vi "RenameVI.vi"(0 "ObjectIn":refnum<class "ClassWriterNative.lvclass">, 1 "VIItemRefIn":refnum<vi>, 2 "RenameOption":T1, 5 "error in (no error)":errorcluster) -> (14 "ObjectOut":refnum<class "ClassWriterNative.lvclass">, 19 "error out":errorcluster)   [LabVIEW 2012, in "ClassWriterNative.lvclass"]
uses:
  <resource>/Framework/Providers/Open_GDS/ClassProviders/Provider_LvNativeClass/ClassWriterNative_class/ClassWriterNative.lvclass
  <resource>/Framework/Providers/Open_GDS/ClassProviders/Provider_BaseClassInterface/ClassWriter_class/RenameViOption.ctl
  <vilib>/picture/picture.llb/imagedata.ctl
  <resource>/Framework/Providers/Open_GDS/ClassProviders/Provider_BaseClassInterface/ClassWriter_class/ClassWriter.lvclass
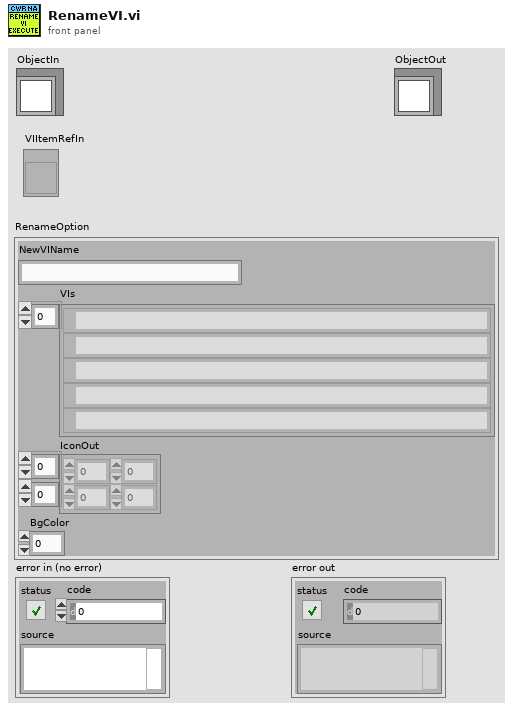
[diagram p1: front panel]
types:
  T1 = typedef "ClassWriter.lvclass/RenameViOption.ctl" = cluster{"NewVIName":string, "VIs":path[], "IconOut":u8[][], "BgColor":u8}
  T2 = cluster{"Counter":i32, "Text":string, "Cancelled":bool, "App Ref":refnum<vi>}
  T3 = typedef "imagedata.ctl" = cluster{"image type":i32, "image depth":i32, "image":u8[], "mask":u8[], "colors":u32[], "Rectangle":cluster{"left":i16, "top":i16, "right":i16, "bottom":i16}}
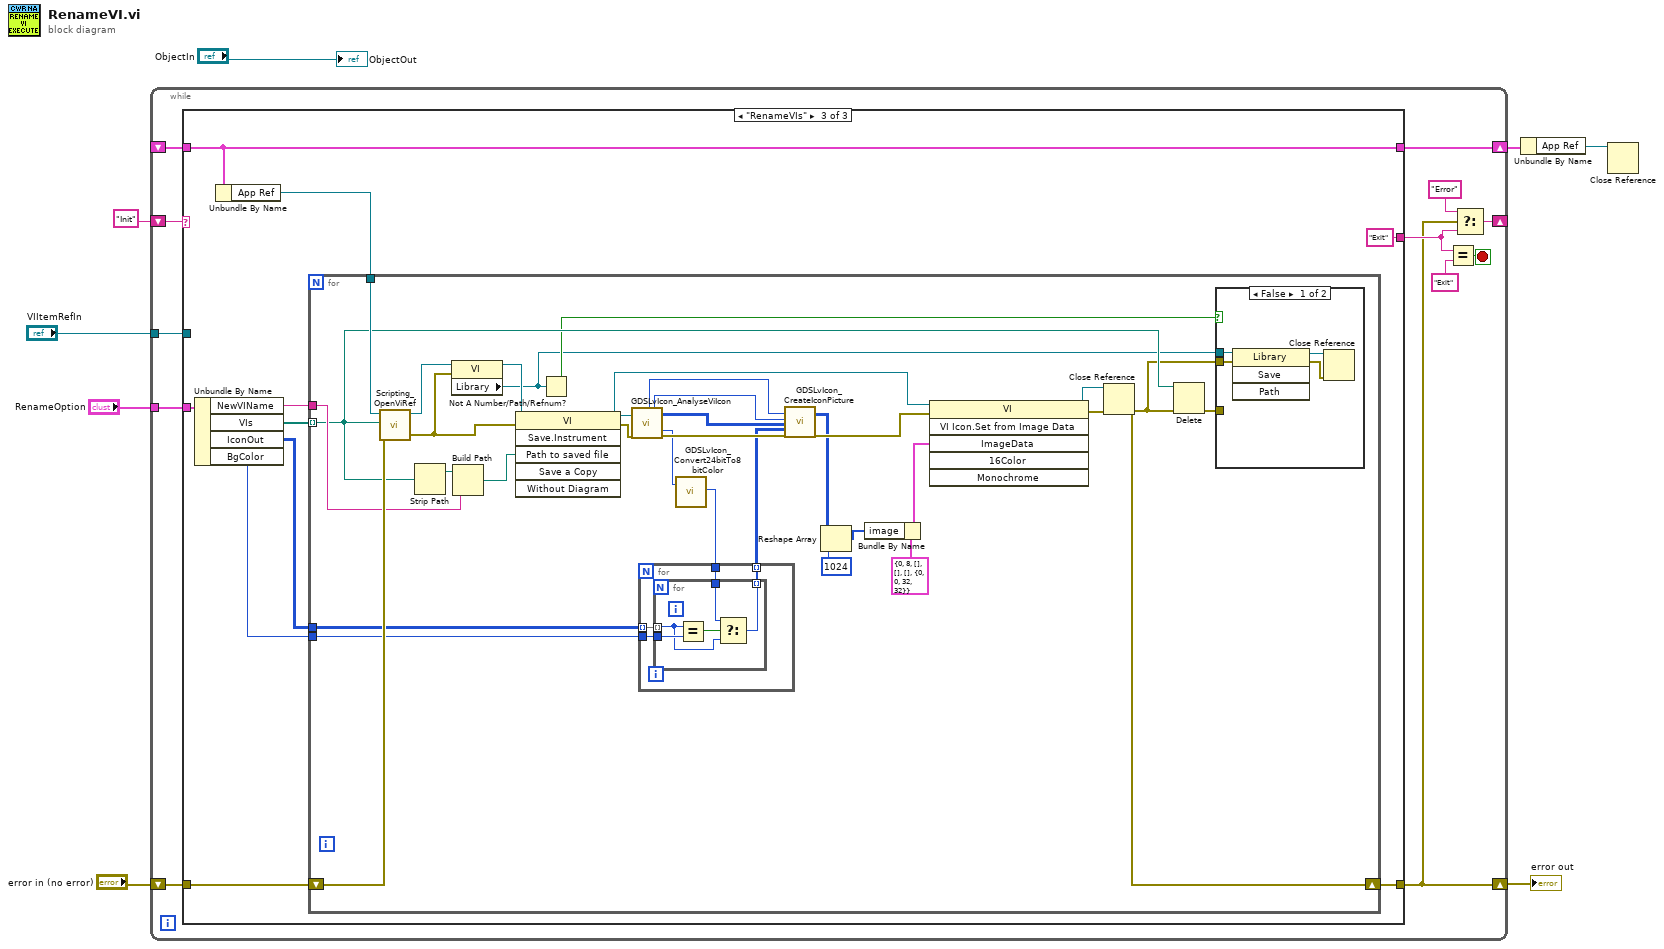
[diagram p0: block diagram]
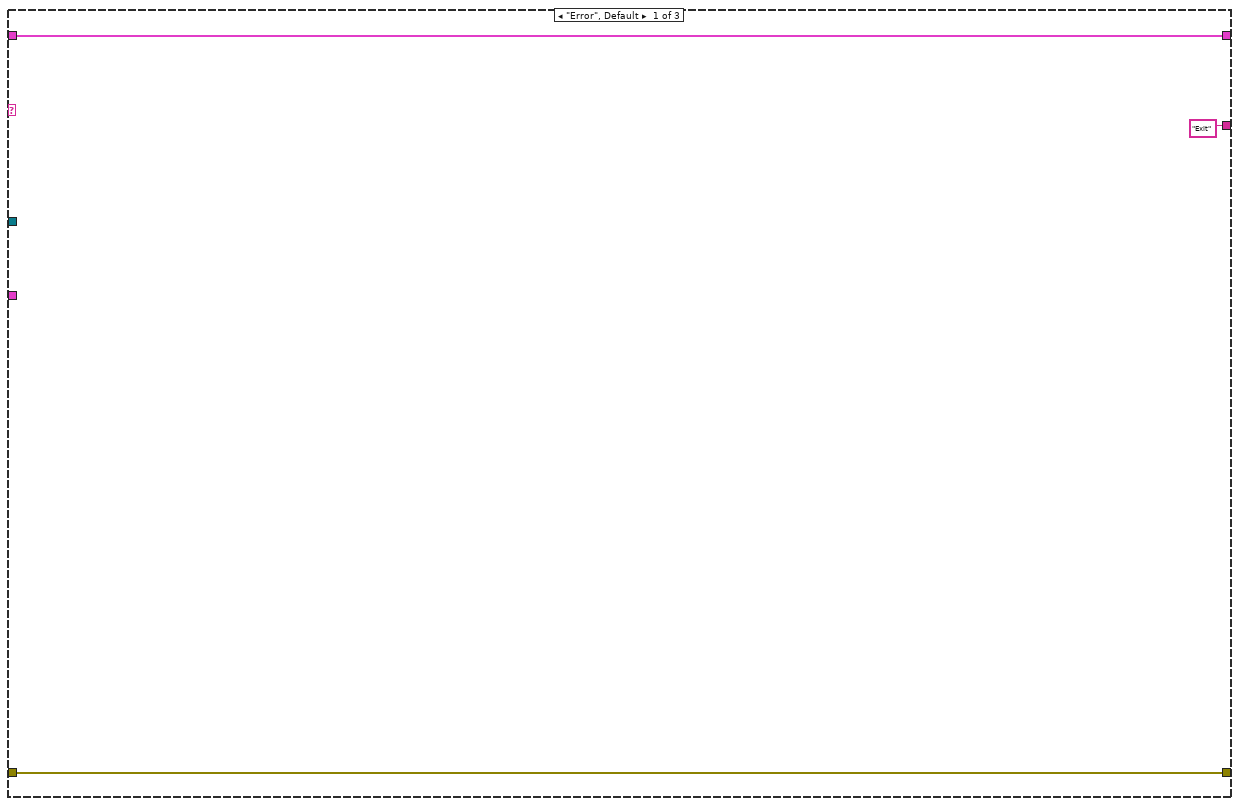
[diagram p2: hidden frame]
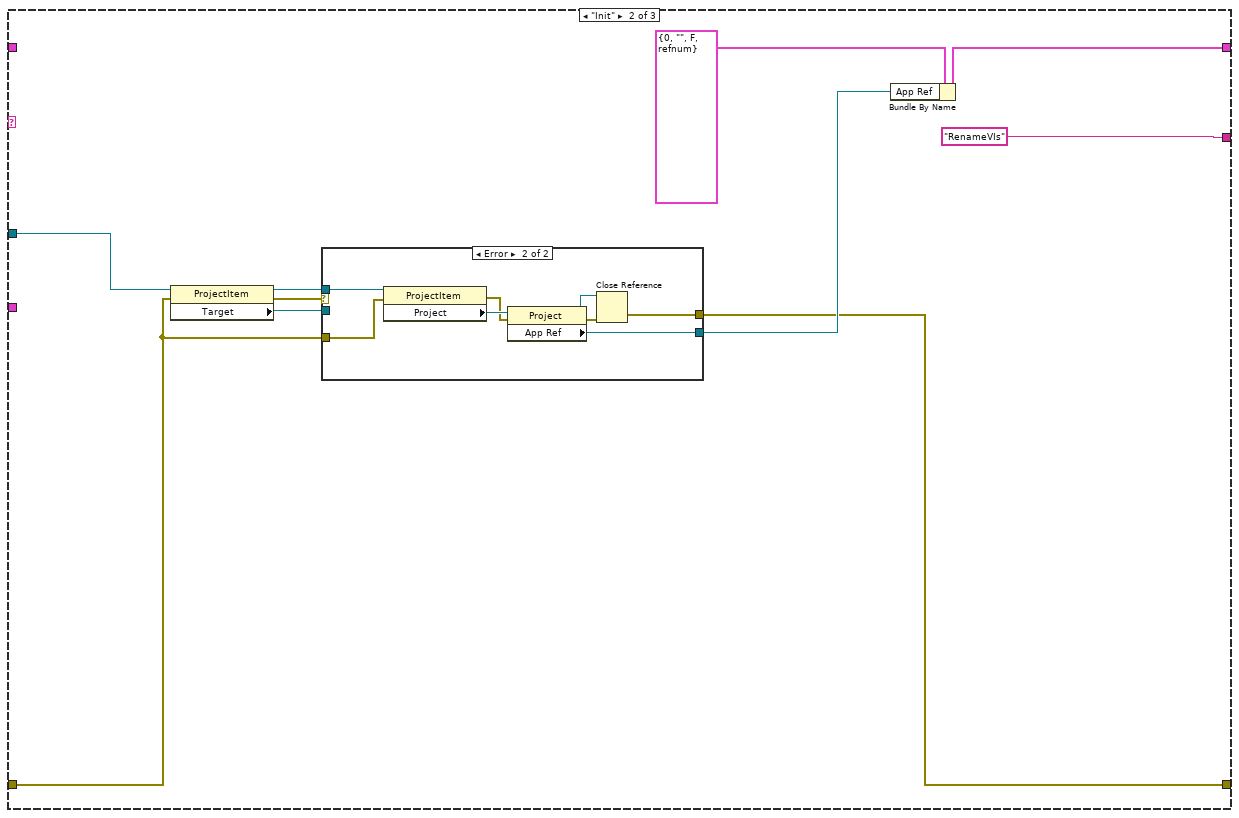
[diagram p3: hidden frame]
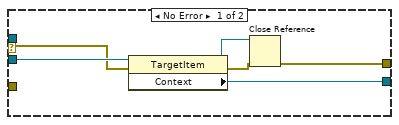
[diagram p4: hidden frame]
diagram:
  n1 = while {
    shift-right: [w13] -> w6
    shift-left: "error in (no error)" -> [w20]
    shift-right: [w18] -> _
    shift-left: "Init" -> [w19]
    shift-right: [w12] -> w8
    shift-left: _ -> [w11]
    tunnel: "RenameOption" -> [w10]
    tunnel: "VIItemRefIn" -> [w9]
    stop <- w17 stop-if-true
    n2 = case shown="\"RenameVIs\"" w19 {
      tunnel: w20 -> [w23 w25 w53]
      tunnel: [w23 w24 w52] -> w13
      tunnel: ["Exit" "RenameVIs" "Exit"] -> w14
      tunnel: [w21 w31 w56] -> w12
      tunnel: w11 -> [w21 _ w56]
      tunnel: w10 -> [_ _ w55]
      tunnel: w9 -> [_ w27 _]
      frame "Error", Default {
      }
      frame "Init" {
        n3 = property class="ProjectItem"(reference=w27, error in=w25) -> (reference out=w28:refnum<vi>, error out=w30:errorcluster, "Target"=w29:refnum<vi>)
        n4 = case shown="Error" w30 {
          selector: w30 -> [w35 _]
          tunnel: w29 -> [w39 _]
          tunnel: [w38 w41] -> w26
          tunnel: [w34 w42] -> w24
          tunnel: w28 -> [_ w47]
          tunnel: w25 -> [_ w46]
          frame No Error {
            n5 = property class="TargetItem"(reference=w39, error in=w35) -> (reference out=w36:refnum<vi>, error out=w37:errorcluster, "Context"=w38:refnum<vi>)
            n6 = Close Reference(reference=w36, error in (no error)=w37) -> (error out=w34:errorcluster)
          }
          frame Error {
            n7 = property class="ProjectItem"(reference=w47, error in=w46) -> (error out=w40:errorcluster, "Project"=w45:refnum<vi>)  [unwired: 1 out]
            n8 = property class="Project"(reference=w45, error in=w40) -> (reference out=w43:refnum<vi>, error out=w44:errorcluster, "App Ref"=w41:refnum<vi>)
            n9 = Close Reference(reference=w43, error in (no error)=w44) -> (error out=w42:errorcluster)
          }
        }
        n10 = Bundle By Name(cluster=T2 {"Counter"=0, "Text"="", "Cancelled"=FALSE, "App Ref"=refnum}, "App Ref"=w26) -> (w31:T2)
      }
      frame "RenameVIs" {
        n11 = Unbundle By Name(w55) -> ("NewVIName"=w51:string, "VIs"=w54:path[], "IconOut"=w50:u8[][], "BgColor"=w49:u8)
        n12 = Unbundle By Name(w56) -> ("App Ref"=w48:refnum<vi>)
        n13 = for {
          tunnel: w54 -> [w65] mode=indexing
          shift-right: [w58] -> w52
          shift-left: w53 -> [w89]
          tunnel: w51 -> [w87]
          tunnel: w50 -> [w75]
          tunnel: w49 -> [w74]
          tunnel: w48 -> [w70]
          n14 = call <resource>:"Scripting_OpenViRef.vi"("error in"=w89, "ViPath/ViName/Viref"=w65, "AppRef"=w70) -> ("error out"=w62:errorcluster, "vi reference"=w64:refnum<vi>)  [unwired: 6 in, 1 out]
          n15 = Strip Path(path=w65) -> (stripped path=w88:path)  [unwired: 1 out]
          n16 = property class="VI"(reference=w64, error in=w62) -> (reference out=w63:refnum<vi>, "Library"=w59:refnum<vi>)  [unwired: 1 out]
          n17 = Build Path(base path=w88, name or relative path=w87) -> (appended path=w86:path)
          n18 = invoke class="VI" method="Save.Instrument"(reference=w63, error in=w62, "Path to saved file"=w86) -> (reference out=w78:refnum<vi>, error out=w85:errorcluster)  [unwired: 3 in, 4 out]
          n19 = Not A Number/Path/Refnum?(number/path/refnum=w59) -> (NaN/Path/Refnum?=w61:bool)
          n20 = call <resource>:"GDSLvIcon_AnalyseViIcon.vi"("ViRef/LvCLassRef/LvLibRef/ViPath"=w78, "error in (no error)"=w85) -> ("FrameColor"=w69:u32, "FrameThickness(1)"=w68:u32, "HeaderIcon"=w76:u8[][], "BodyBkColor"=w72:u32, "error out"=w84:errorcluster)  [unwired: 5 in, 8 out]
          n21 = call <resource>:"GDSLvIcon_Convert24bitTo8bitColor.vi"("Color 24bit In"=w72) -> ("Color out(256)"=w71:u8)  [unwired: 15 in, 3 out]
          n22 = for {
            tunnel: w75 -> [w97] mode=indexing
            tunnel: w71 -> [w96]
            tunnel: w74 -> [w95]
            tunnel: [w94] -> w73 mode=indexing
            n23 = for {
              tunnel: w97 -> [w98] mode=indexing
              tunnel: w96 -> [w101]
              tunnel: w95 -> [w99]
              tunnel: [w100] -> w94 mode=indexing
              n24 = Equal?(x=w98, y=w99) -> (x = y?=w102:bool)
              n25 = Select(t=w101, s=w102, f=w98) -> (s? t:f=w100:u8)
            }
          }
          n26 = call <resource>:"GDSLvIcon_CreateIconPicture.vi"("FrameColor"=w69, "FrameThickness(1)"=w68, "HeaderIconIn"=w76, "BodyIconIn"=w73, "error in (no error)"=w84) -> ("WholeIconOut"=w77:u8[][], "error out"=w79:errorcluster)  [unwired: 9 in, 4 out]
          n27 = Reshape Array(w77, 1024 ("dimension size")) -> (w80:u8[])
          n28 = Bundle By Name(cluster=T3 {"image type"=0, "image depth"=8, "image"=[], "mask"=[], "colors"=[], "Rectangle"={"left"=0, "top"=0, "right"=32, "bottom"=32}} ("image data"), "image"=w80) -> (w81:T3)
          n29 = invoke class="VI" method="VI Icon.Set from Image Data"(reference=w78, error in=w79, "ImageData"=w81) -> (reference out=w66:refnum<vi>, error out=w67:errorcluster)  [unwired: 3 in, 4 out]
          n30 = Close Reference(reference=w66, error in (no error)=w67) -> (error out=w58:errorcluster)
          n31 = Delete(path (use dialog)=w65, error in=w58) -> (error out=w60:errorcluster)  [unwired: 3 in, 2 out]
          n32 = case shown="False" w61 {
            tunnel: w60 -> [_ _]
            tunnel: w59 -> [w93 _]
            tunnel: w58 -> [w92 _]
            frame False {
              n33 = invoke class="Library" method="Save"(reference=w93, error in=w92) -> (reference out=w91:refnum<vi>, error out=w90:errorcluster)  [unwired: 2 in, 2 out]
              n34 = Close Reference(reference=w91, error in (no error)=w90) -> ()  [unwired: 1 out]
            }
            frame True {
            }
          }
        }
      }
    }
    n35 = Equal?(x=w14, y="Exit") -> (x = y?=w17:bool)
    n36 = Select(t="Error", s=w13, f=w14) -> (s? t:f=w18:string)
  }
  "error out" <- w6
  n37 = Unbundle By Name(w8) -> ("App Ref"=w1:refnum<vi>)
  n38 = Close Reference(reference=w1) -> ()  [unwired: 1 in, 1 out]
  "ObjectOut" <- "ObjectIn"
